vi "GLdrv_FILE_LIST.vi"(0 "Connection ID":T1, 11 "error in (no error)":errorcluster) -> (4 "Connection ID Out":T1, 6 "File List":string[](array[string]), 15 "error out":errorcluster)   [LabVIEW 2017, in "GL860_Driver.lvlib"]
doc: "CDで設定されているカレントパス内のファイルをリスト表示します"
uses:
  GL860_Driver.lvlib
  ConnectionID.ctl
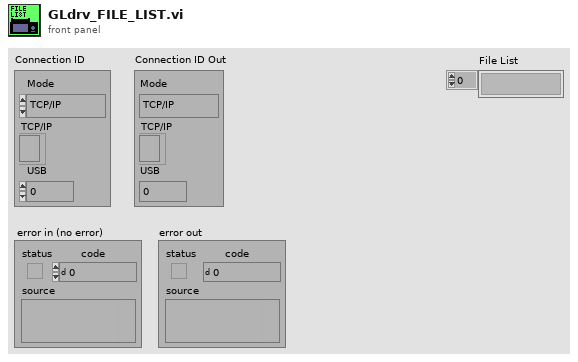
[diagram p1: front panel]
types:
  T1 = typedef "ConnectionID.ctl" = cluster{"Mode":enum16{"TCP/IP", "USB"}, "TCP/IP":refnum<k5>, "USB":i32}
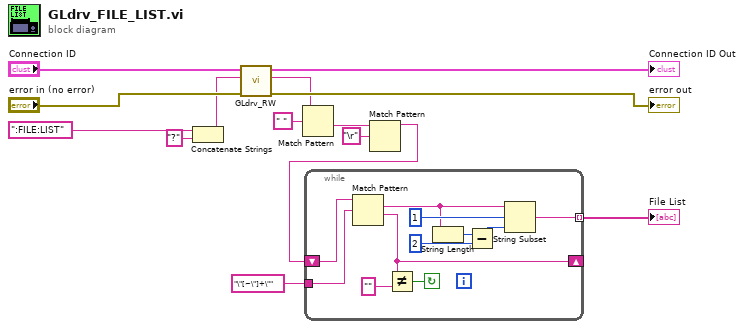
[diagram p0: block diagram]
diagram:
  n1 = Concatenate Strings(":FILE:LIST" ("Command"), "?" ("string")) -> (w4:string)
  n2 = call "GLdrv_RW.vi"("error in (no error)"="error in (no error)", "data in"=w4, "Connection ID"="Connection ID") -> ("error out"=→"error out":errorcluster, "data out"=w3:string, "Connection ID Out"=→"Connection ID Out":T1)  [unwired: 4 in, 2 out]
  n3 = Match Pattern(string=w3, regular expression=" " ("search string/char (-)")) -> (after substring=w6:string)  [unwired: 4 out]
  n4 = Match Pattern(string=w6, regular expression="\r") -> (before substring=w2:string)  [unwired: 4 out]
  n5 = while {
    tunnel: [w16] -> w9 mode=indexing
    shift-right: [w24] -> _
    shift-left: w2 -> [w25]
    tunnel: "\"[~\"]+\"" ("regular expression") -> [w15]
    stop <- w22 continue-if-true
    n6 = Match Pattern(string=w25, regular expression=w15) -> (match substring=w17:string, after substring=w24:string)  [unwired: 3 out]
    n7 = Not Equal?(x=w24, y="") -> (x != y?=w22:bool)
    n8 = String Length(string=w17) -> (length=w19:i32)
    n9 = Subtract(x=w19, y=2) -> (x-y=w20:i32)
    n10 = String Subset(string=w17, offset (0)=1, length (rest)=w20) -> (substring=w16:string)
  }
  "File List" <- w9
